vi "DrawTriangle.vi"(6 "Open?":bool, 7 "Collection in":refnum<class "Collection.lvclass">, 8 "error in":errorcluster, 9 "Point":refnum<class "Point.lvclass">, 10 "Color":refnum<class "Color.lvclass">, 11 "Menu in":refnum<class "Menu.lvclass">) -> (0 "error out":errorcluster, 3 "Menu out":refnum<class "Menu.lvclass">, 5 "Collection out":refnum<class "Collection.lvclass">)   [LabVIEW 2021, in "Menu.lvlib" / "Menu.lvclass"]
uses:
  Menu.lvclass
  Menu.lvclass/Menu.ctl
  Picture2D/src/TriangleR/TriangleR.lvclass
  Picture2D/src/Line/Line.lvclass
  Picture2D/src/Collection/Collection.lvclass
  Picture2D/src/Point/Point.lvclass
  Picture2D/src/Picture2D/Picture2D.lvclass
  C:/GitHub/Picture2D/src/Triangle/Triangle.lvclass
  C:/GitHub/Picture2D/src/Polygone/Polygone.lvclass
  C:/GitHub/Picture2D/src/Shape/Shape.lvclass
  C:/GitHub/Picture2D/src/Picture2D/Picture2D.lvclass
  C:/GitHub/Picture2D/src/IDrawable/IDrawable.lvclass
  C:/GitHub/Picture2D/src/IMovable/IMovable.lvclass
  C:/GitHub/Picture2D/src/IRotatable/IRotatable.lvclass
  C:/GitHub/Picture2D/src/IScalable/IScalable.lvclass
  C:/GitHub/Picture2D/src/TriangleR/TriangleR.lvclass
  C:/GitHub/Picture2D/src/Line/Line.lvclass
  Picture2D/src/Color/Color.lvclass
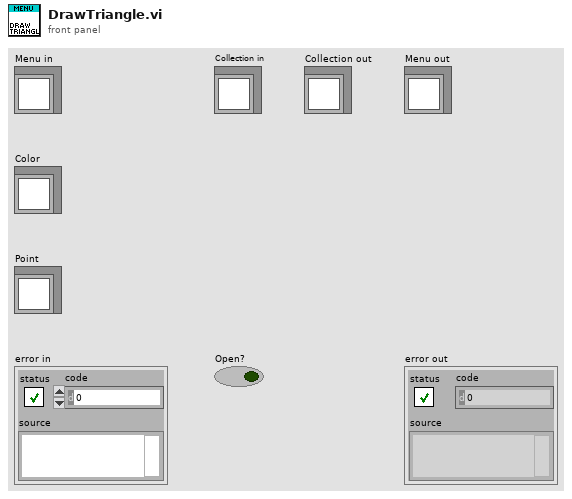
[diagram p1: front panel]
types:
  T1 = typedef "Menu.lvlib/Menu.lvclass/SubMenuIcon.ctl" = enum16{"LabVIEW", "Windows", "Custom"}
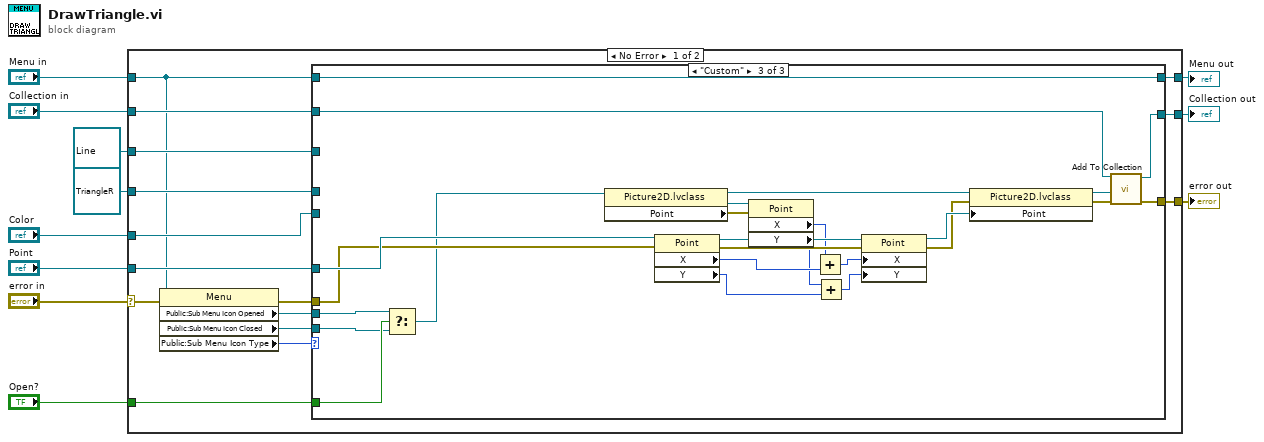
[diagram p0: block diagram]
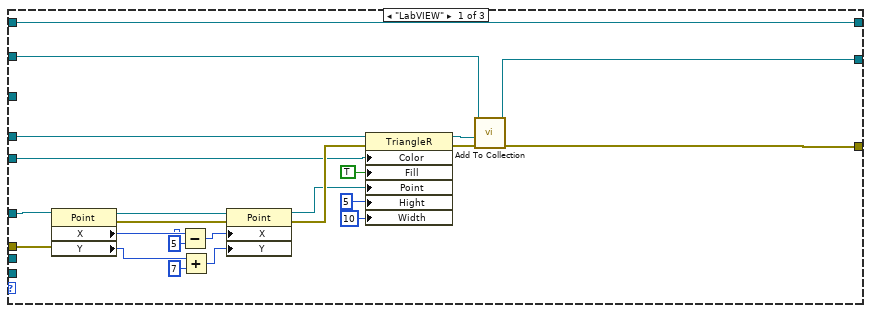
[diagram p2: hidden frame]
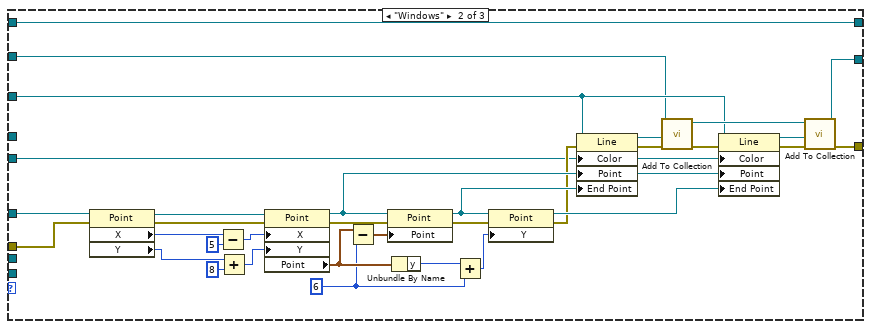
[diagram p3: hidden frame]
diagram:
  n1 = case shown="No Error" "error in" {
    selector: "error in" -> [w17 w110]
    tunnel: [w25 w110] -> w11
    tunnel: "Point" -> [w21 _]
    tunnel: "Color" -> [w20 _]
    tunnel: refnum<class "TriangleR.lvclass"> refnum ("Triangle") -> [w26 _]
    tunnel: refnum<class "Line.lvclass"> refnum ("Line") -> [w22 _]
    tunnel: "Collection in" -> [w23 w109]
    tunnel: [w24 w109] -> w1
    tunnel: "Open?" -> [w19 _]
    tunnel: "Menu in" -> [w15 w108]
    tunnel: [w18 w108] -> w3
    frame No Error {
      n2 = property class="Menu"(reference=w15, error in=w17) -> (error out=w16:errorcluster, "Public:Sub Menu Icon Opened"=w12:refnum<class "Picture2D.lvclass">, "Public:Sub Menu Icon Closed"=w14:refnum<class "Picture2D.lvclass">, "Public:Sub Menu Icon Type"=w13:T1)  [unwired: 1 out]
      n3 = case shown="\"Custom\"" w13 {
        tunnel: w23 -> [w39 w53 w105]
        tunnel: w16 -> [w36 w51 w93]
        tunnel: w26 -> [w35 _ _]
        tunnel: [w31 w55 w107] -> w25
        tunnel: [w30 w54 w106] -> w24
        tunnel: w22 -> [_ w56 _]
        tunnel: w21 -> [w29 w57 w95]
        tunnel: w20 -> [w28 w52 _]
        tunnel: w19 -> [_ _ w87]
        tunnel: w14 -> [_ _ w86]
        tunnel: w15 -> [w27 w50 w84]
        tunnel: [w27 w50 w84] -> w18
        tunnel: w12 -> [_ _ w83]
        frame "LabVIEW" {
          n4 = property class="Point"(reference=w29, error in=w36) -> (reference out=w40:refnum<class "Point.lvclass">, error out=w43:errorcluster, "X"=w47:i16, "Y"=w46:i16)
          n5 = Subtract(x=w47, y=i16 5) -> (x-y=w42:i16)
          n6 = Add(x=w46, y=i16 7) -> (x+y=w41:i16)
          n7 = property class="Point"(reference=w40, error in=w43, "X"=w42, "Y"=w41) -> (reference out=w44:refnum<class "Point.lvclass">, error out=w45:errorcluster)
          n8 = property class="TriangleR"(reference=w35, error in=w45, "Color"=w28, "Fill"=TRUE, "Point"=w44, "Hight"=i16 5, "Width"=i16 10) -> (reference out=w49:refnum<class "TriangleR.lvclass">, error out=w48:errorcluster)
          n9 = call-dynamic "Add To Collection.vi"("error in (no error)"=w48, "IDrawable"=w49, "Collection in"=w39) -> ("error out"=w31:errorcluster, "Collection out"=w30:refnum<class "Collection.lvclass">)  [unwired: 7 in]
        }
        frame "Windows" {
          w60 = i16 6
          n10 = property class="Point"(reference=w57, error in=w51) -> (reference out=w61:refnum<class "Point.lvclass">, error out=w64:errorcluster, "X"=w66:i16, "Y"=w65:i16)
          n11 = Subtract(x=w66, y=i16 5) -> (x-y=w63:i16)
          n12 = Add(x=w65, y=i16 8) -> (x+y=w62:i16)
          n13 = property class="Point"(reference=w61, error in=w64, "X"=w63, "Y"=w62) -> (reference out=w77:refnum<class "Point.lvclass">, error out=w67:errorcluster, "Point"=w81:cluster{"x":i16, "y":i16})
          n14 = Subtract(x=w81, y=w60) -> (x-y=w79:cluster{"x":i16, "y":i16})
          n15 = property class="Point"(reference=w77, error in=w67, "Point"=w79) -> (reference out=w78:refnum<class "Point.lvclass">, error out=w74:errorcluster)
          n16 = Unbundle By Name(w81) -> ("y"=w82:i16)
          n17 = Add(x=w82, y=w60) -> (x+y=w80:i16)
          n18 = property class="Point"(reference=w78, error in=w74, "Y"=w80) -> (reference out=w76:refnum<class "Point.lvclass">, error out=w75:errorcluster)
          n19 = property class="Line"(reference=w56, error in=w75, "Color"=w52, "Point"=w77, "End Point"=w78) -> (reference out=w70:refnum<class "Line.lvclass">, error out=w68:errorcluster)
          n20 = call-dynamic "Add To Collection.vi"("error in (no error)"=w68, "IDrawable"=w70, "Collection in"=w53) -> ("error out"=w69:errorcluster, "Collection out"=w73:refnum<class "Collection.lvclass">)  [unwired: 7 in]
          n21 = property class="Line"(reference=w56, error in=w69, "Color"=w52, "Point"=w77, "End Point"=w76) -> (reference out=w72:refnum<class "Line.lvclass">, error out=w71:errorcluster)
          n22 = call-dynamic "Add To Collection.vi"("error in (no error)"=w71, "IDrawable"=w72, "Collection in"=w73) -> ("error out"=w55:errorcluster, "Collection out"=w54:refnum<class "Collection.lvclass">)  [unwired: 7 in]
        }
        frame "Custom" {
          n23 = Select(t=w83, s=w87, f=w86) -> (s? t:f=w85:refnum<class "Picture2D.lvclass">)
          n24 = property class="Picture2D.lvclass"(reference=w85) -> (reference out=w92:refnum<class "Picture2D.lvclass">, error out=w90:errorcluster, "Point"=w91:refnum<class "Point.lvclass">)  [unwired: 1 in]
          n25 = property class="Point"(reference=w95, error in=w93) -> (reference out=w97:refnum<class "Point.lvclass">, error out=w100:errorcluster, "X"=w102:i16, "Y"=w101:i16)
          n26 = property class="Point"(reference=w91, error in=w90) -> ("X"=w89:i16, "Y"=w88:i16)  [unwired: 2 out]
          n27 = Add(x=w89, y=w102) -> (x+y=w99:i16)
          n28 = Add(x=w88, y=w101) -> (x+y=w98:i16)
          n29 = property class="Point"(reference=w97, error in=w100, "X"=w99, "Y"=w98) -> (reference out=w96:refnum<class "Point.lvclass">, error out=w94:errorcluster)
          n30 = property class="Picture2D.lvclass"(reference=w92, error in=w94, "Point"=w96) -> (reference out=w103:refnum<class "Picture2D.lvclass">, error out=w104:errorcluster)
          n31 = call-dynamic "Add To Collection.vi"("error in (no error)"=w104, "IDrawable"=w103, "Collection in"=w105) -> ("error out"=w107:errorcluster, "Collection out"=w106:refnum<class "Collection.lvclass">)  [unwired: 7 in]
        }
      }
    }
    frame Error {
    }
  }
  "error out" <- w11
  "Menu out" <- w3
  "Collection out" <- w1
